vi "Set-camera-menu.vi"(7 "Menu ref.":refnum<k9>, 8 "error in (no error)":errorcluster, 10 "Camera in":T1, 11 "UI ref. in":refnum<data-value>) -> (0 "error out":errorcluster, 3 "UI ref.":refnum<data-value>)   [LabVIEW 2013, in "CameraVision.lvlib" / "CV-UI.lvclass"]
uses:
  CV-UI.lvclass
  Camera-selector.ctl
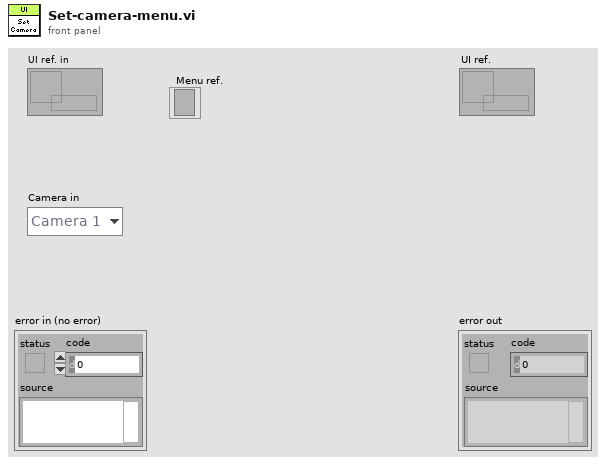
[diagram p1: front panel]
types:
  T1 = typedef "CameraVision.lvlib/CV-UI.lvclass/Camera-selector.ctl" = enum16{"Camera 1", "Camera 2"}
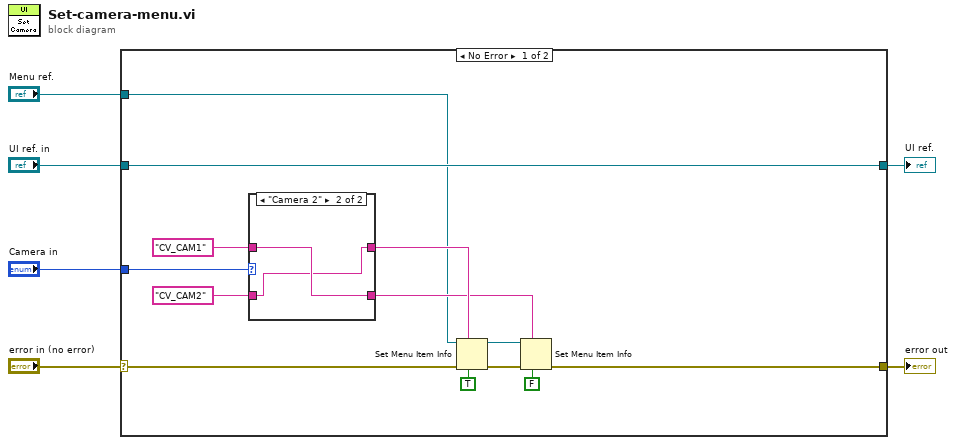
[diagram p0: block diagram]
diagram:
  n1 = case shown="No Error" "error in (no error)" {
    selector: "error in (no error)" -> [w12 w25]
    tunnel: [w9 w25] -> w5
    tunnel: "UI ref. in" -> [w8 w24]
    tunnel: [w8 w24] -> w3
    tunnel: "Camera in" -> [w15 _]
    tunnel: "Menu ref." -> [w7 _]
    frame No Error {
      n2 = case shown="\"Camera 2\"" w15 {
        tunnel: "CV_CAM1" ("item tag") -> [w20 w23]
        tunnel: "CV_CAM2" ("item tag") -> [w21 w22]
        tunnel: [w21 w23] -> w10
        tunnel: [w20 w22] -> w11
        frame "Camera 1", Default {
        }
        frame "Camera 2" {
        }
      }
      n3 = Set Menu Item Info(6:TRUE ("checked"), 7:w11, 8:w12, 11:w7) -> (0:w16:errorcluster, 3:w19:refnum<k9>)  [unwired: 3 in]
      n4 = Set Menu Item Info(6:FALSE ("checked"), 7:w10, 8:w16, 11:w19) -> (0:w9:errorcluster)  [unwired: 3 in, 1 out]
    }
    frame Error {
    }
  }
  "error out" <- w5
  "UI ref." <- w3
